vi "Global Variables.vi"() -> ()   [LabVIEW 2011]
panel:
  in  "Gains":T1={"Proportional Gain"=20, "Integral Gain"=10, "Derivative Gain"=0}
  out "Rate (usec)":u32
  out "PWM Index 3":i16
  out "PWM Index 2":i16
  out "PWM Index 1":i16
  out "PWM Redundant":i16
  out "PWM Middle 3":i16
  out "PWM Middle 2":i16
  out "PWM Middle 1":i16
  out "PWM Thumb 3":i16
  out "PWM Thumb 2":i16
  out "Trigger Redundant":bool
  out "Trigger Index 3":bool
  out "Trigger Index 2":bool
  out "Trigger Index 1":bool
  out "Trigger Middle 3":bool
  out "Trigger Middle 2":bool
  out "Trigger Middle 1":bool
  out "Trigger Thumb 3":bool
  out "Trigger Thumb 2":bool
  out "PWM Thumb 1":i16
  out "Trigger Thumb 1":bool
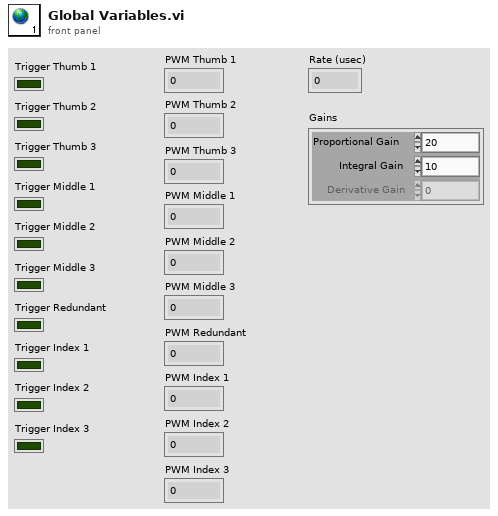
[diagram p1: front panel]
types:
  T1 = cluster{"Proportional Gain":i16, "Integral Gain":i16, "Derivative Gain":i16}
diagram:
